vi "Get Frame Array File Path.vi"(8 "error in":errorcluster, 11 "custom device ref in":T1 format="%.0x") -> (0 "error out":errorcluster, 1 "MD5 checksum":string, 2 "Frame Array File Path":path, 3 "custom device ref out":T1 format="%.0x", 4 "Found?":bool)   [LabVIEW 2020, in "AIM ARINC 664 Scripting.lvlib"]
uses:
  AIM ARINC 664 Scripting.lvlib
  <vilib>/NI VeriStand/Custom Device API/Custom Device API.lvlib
  Constants.vi
  <vilib>/NI VeriStand/Custom Device API/Get Item Property (Dependent File).vi
  <vilib>/NI VeriStand/Custom Device Tools/Custom Device Utility Library/Custom Device Utility Library.lvlib
  <vilib>/NI VeriStand/Custom Device Tools/Custom Device Utility Library/NI VeriStand - Search for Item by GUID.vi
  <vilib>/NI VeriStand/Custom Device API/Custom Device Item Ref.ctl
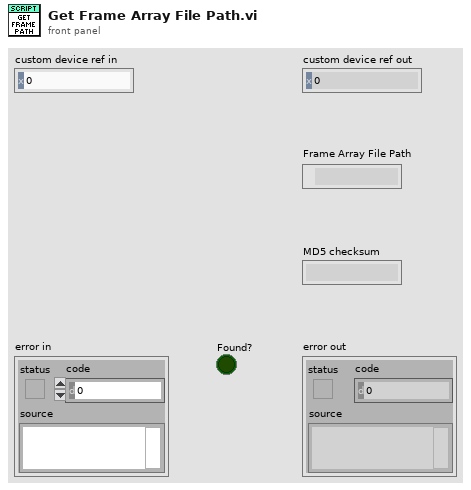
[diagram p1: front panel]
types:
  T1 = typedef "Custom Device API.lvlib/Custom Device Item Ref.ctl" = u64
  T2 = typedef "Custom Device API.lvlib/Dependent File Optional Info.ctl" = cluster{"Version":string, "RTDestination":path, "ForceDownload":bool, "SupportedTarget":string, "MD5":string}
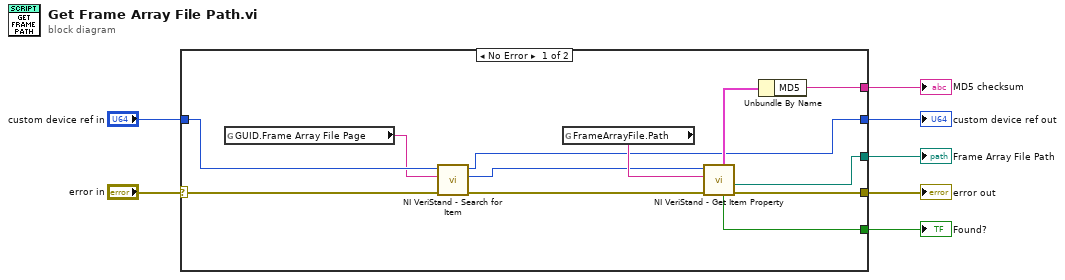
[diagram p0: block diagram]
diagram:
  n1 = case shown="No Error" "error in" {
    selector: "error in" -> [w12 w21]
    tunnel: "custom device ref in" -> [w17 w20]
    tunnel: [w19 w21] -> w6
    tunnel: [w8 w20] -> w5
    tunnel: [w16 _] -> w3
    tunnel: [w15 _] -> w2
    tunnel: [w13 _] -> w1
    frame No Error {
      n2 = global read "Constants.vi" "GUID.Frame Array File Page"() -> (w10:string)
      n3 = call-poly <vilib>:"NI VeriStand - Search for Item.vi"("error in"=w12, "Item GUID"=w10, "Section Ref in"=w17) -> ("error out"=w11:errorcluster, "Item Ref"=w9:T1, "Section Ref out"=w8:T1)  [unwired: 5 in, 1 out]
      n4 = global read "Constants.vi" "FrameArrayFile.Path"() -> (w18:string)
      n5 = call-poly <vilib>:"NI VeriStand - Get Item Property.vi"("error in (no error)"=w11, "Property Name"=w18, "Item Ref in"=w9) -> ("error out"=w19:errorcluster, "Path"=w16:path, "Found"=w15:bool, "OptionalInfo"=w14:T2)  [unwired: 4 in, 1 out]
      n6 = Unbundle By Name(w14) -> ("MD5"=w13:string)
    }
    frame Error {
    }
  }
  "error out" <- w6
  "Frame Array File Path" <- w3
  "custom device ref out" <- w5
  "Found?" <- w2
  "MD5 checksum" <- w1
